vi "tables.vi"(0 "report in":refnum<class "NI_Standard Report.lvclass">, 1 "show grid lines":bool, 2 "column width":dbl=1.0 format="%.2f", 5 "column headers":string[](array[string]), 9 "row headers":string[](array[string]), 11 "error in (no error)":errorcluster, 12 "text data":string[][](array[string]), 13 "Measurement System":i32) -> (4 "report out":refnum<class "NI_Standard Report.lvclass">, 15 "error out":errorcluster)   [LabVIEW 2015, in "NI_Standard Report.lvclass"]
uses:
  <vilib>/Utility/NIReport.llb/Standard Report/NI_Standard Report.lvclass
  <vilib>/Utility/NIReport.llb/Standard Report/NI_Standard Report.lvclass/NI_Standard Report.ctl
  <vilib>/Utility/NIReport.llb/NI_ReportGenerationCore.lvlib
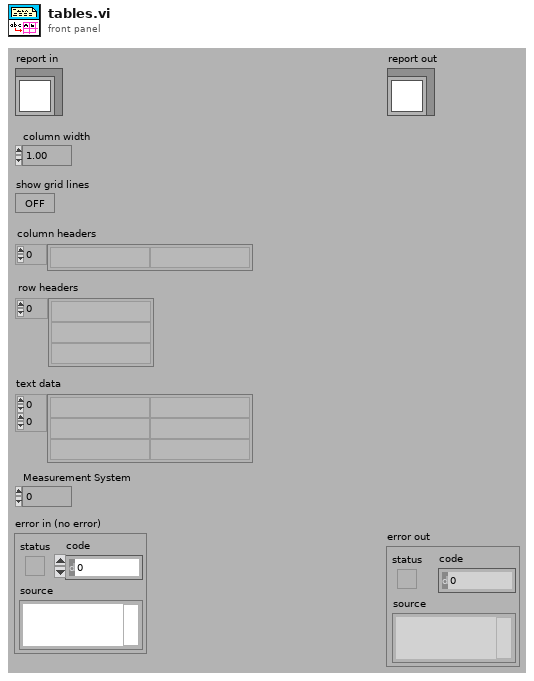
[diagram p1: front panel]
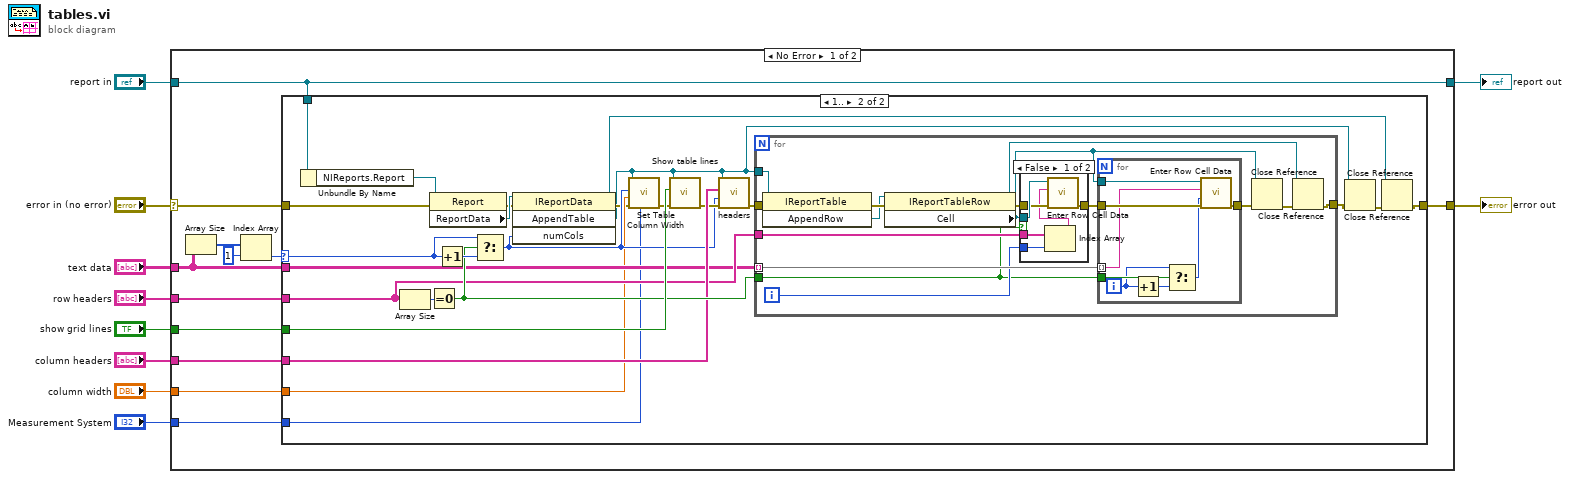
[diagram p0: block diagram]
diagram:
  n1 = case shown="No Error" "error in (no error)" {
    selector: "error in (no error)" -> [w14 w80]
    tunnel: [w13 w80] -> w9
    tunnel: [w18 w79] -> w7
    tunnel: "report in" -> [w18 w79]
    tunnel: "text data" -> [w20 _]
    tunnel: "row headers" -> [w17 _]
    tunnel: "show grid lines" -> [w16 _]
    tunnel: "column headers" -> [w15 _]
    tunnel: "column width" -> [w12 _]
    tunnel: "Measurement System" -> [w11 _]
    frame No Error {
      n2 = Array Size(array=w20) -> (size(s)=w21:i32[])
      n3 = Index Array(array=w21, index=1 ("Index")) -> (element=w19:i32)
      n4 = case shown="1.." w19 {
        selector: w19 -> [_ w27]
        tunnel: w16 -> [_ w46]
        tunnel: w15 -> [_ w41]
        tunnel: w17 -> [_ w40]
        tunnel: w20 -> [_ w39]
        tunnel: w14 -> [w23 w24]
        tunnel: w12 -> [_ w35]
        tunnel: w11 -> [_ w26]
        tunnel: [w23 w29] -> w13
        tunnel: w18 -> [_ w25]
        frame 0, Default {
        }
        frame 1.. {
          n5 = Unbundle By Name(w25) -> ("NIReports.Report"=w38:refnum<k7>)
          n6 = Array Size(array=w40) -> (size(s)=w45:i32)
          n7 = Equal To 0?(x=w45) -> (x = 0?=w42:bool)
          n8 = property class="Report"(reference=w38, error in=w24) -> (error out=w47:errorcluster, "ReportData"=w48:refnum<k7>)  [unwired: 1 out]
          n9 = Increment(x=w27) -> (x+1=w43:i32)
          n10 = Select(t=w27, s=w42, f=w43) -> (s? t:f=w36:i32)
          n11 = invoke class="IReportData" method="AppendTable"(reference=w48, error in=w47, "numCols"=w36) -> (reference out=w28:refnum<k7>, error out=w34:errorcluster, "AppendTable"=w32:refnum<k7>)  [unwired: 1 in, 1 out]
          n12 = call <vilib>:"Set Table Column Width.vi"("MeasurementSystem"=w26, "error in"=w34, "Column Width"=w35, "Number of Columns"=w36, "AppendTable"=w32) -> ("error out"=w33:errorcluster)  [unwired: 6 out]
          n13 = call <vilib>:"Show table lines.vi"("error in"=w33, "Show Table Lines"=w46, "AppendTable"=w32) -> ("error out"=w37:errorcluster)  [unwired: 8 out]
          n14 = call <vilib>:"headers.vi"("error in"=w37, "Number of Columns"=w36, "Column Headers"=w41, "AppendTable"=w32) -> ("error out"=w44:errorcluster)  [unwired: 7 out]
          n15 = for {
            tunnel: w39 -> [w63] mode=indexing
            tunnel: w32 -> [w60]
            tunnel: w44 -> [w61]
            tunnel: w40 -> [w59]
            tunnel: w42 -> [w55]
            tunnel: [w51] -> w31
            i -> [w58]
            n16 = invoke class="IReportTable" method="AppendRow"(reference=w60, error in=w61) -> (error out=w62:errorcluster, "AppendRow"=w54:refnum<k7>)  [unwired: 1 in, 1 out]
            n17 = property class="IReportTableRow"(reference=w54, error in=w62) -> (reference out=w49:refnum<k7>, error out=w57:errorcluster, "Cell"=w50:refnum<k7>)
            n18 = case shown="False" w55 {
              tunnel: w59 -> [w69 _]
              tunnel: w58 -> [w68 _]
              tunnel: w50 -> [w67 _]
              tunnel: w57 -> [w66 w70]
              tunnel: [w65 w70] -> w56
              frame False {
                n19 = Index Array(array=w69, index=w68) -> (element=w64:string)
                n20 = call <vilib>:"Enter Row Cell Data.vi"("error in (no error)"=w66, "text"=w64, "cell"=w67) -> ("error out"=w65:errorcluster)  [unwired: 1 in, 7 out]
              }
              frame True {
              }
            }
            n21 = for {
              tunnel: w50 -> [w75]
              tunnel: w63 -> [w77] mode=indexing
              tunnel: w56 -> [w78]
              tunnel: [w76] -> w52
              tunnel: w55 -> [w73]
              i -> [w72]
              n22 = Increment(x=w72) -> (x+1=w74:i32)
              n23 = Select(t=w72, s=w73, f=w74) -> (s? t:f=w71:i32)
              n24 = call <vilib>:"Enter Row Cell Data.vi"("error in (no error)"=w78, "row index"=w71, "text"=w77, "cell"=w75) -> ("error out"=w76:errorcluster)  [unwired: 7 out]
            }
            n25 = Close Reference(reference=w50, error in (no error)=w52) -> (error out=w53:errorcluster)
            n26 = Close Reference(reference=w49, error in (no error)=w53) -> (error out=w51:errorcluster)
          }
          n27 = Close Reference(reference=w32, error in (no error)=w31) -> (error out=w30:errorcluster)
          n28 = Close Reference(reference=w28, error in (no error)=w30) -> (error out=w29:errorcluster)
        }
      }
    }
    frame Error {
    }
  }
  "error out" <- w9
  "report out" <- w7
